vi "SAC-Read Responses.vi"(2 "State":T1, 7 "filestem":string, 11 "error in (no error)":errorcluster) -> (6 "time":cluster{"offset":dbl, "dx":dbl, "Y":dbl[]}, 8 "crosscorr":cluster{"offset":dbl, "dx":dbl, "Y":dbl[]}, 13 "phase":cluster{"offset":dbl, "dx":dbl, "Y":dbl[]}, 14 "mag":cluster{"offset":dbl, "dx":dbl, "Y":dbl[]}, 15 "error out":errorcluster)   [LabVIEW 2020]
uses:
  Typedefs/SAC-State.ctl
  <vilib>/Analysis/2dsp.llb/Complex FFT.vi
  <vilib>/Analysis/2dsp.llb/Inverse Real FFT.vi
  Utility VIs/Math VIs/FFT x(t) to dB,Degrees (1D).vi
  Utility VIs/Conversion VIs/Create Waveform Cluster (1D).vi
  <vilib>/Analysis/NI_AALPro.lvlib
panel:
  out "error out":errorcluster
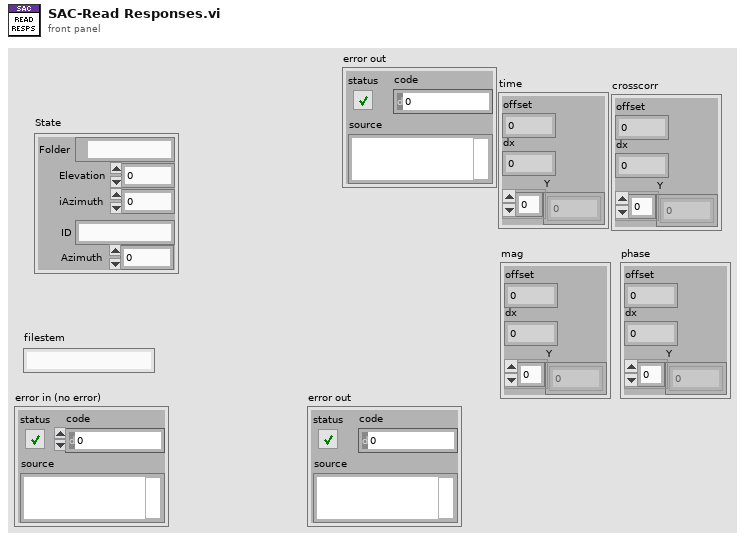
[diagram p1: front panel]
types:
  T1 = typedef "SAC-State.ctl" = cluster{"Folder":path, "Elevation":dbl, "iAzimuth":i32, "ID":string, "Azimuth":dbl}
  T2 = typedef "SAC-Parameters.ctl" = cluster{"Fs (Hz)":dbl, "atten (dB)":dbl, "Waveform":T3, "Freq Res (Hz)":dbl, "Order":i32, "Averages":i32, "seed":i64, "Window":T4, "Mic gain":dbl, "Mic sens":dbl}
  T3 = typedef "HRTF-Waveform.ctl" = enum16{"Chirp", "MLS"}
  T4 = typedef "HRTF-Window.ctl" = cluster{"Type":T5, "Length (ms)":dbl, "Center (ms)":dbl}
  T5 = typedef "HRTF-Window Type.ctl" = enum16{"None", "Rectangle", "Hanning"}
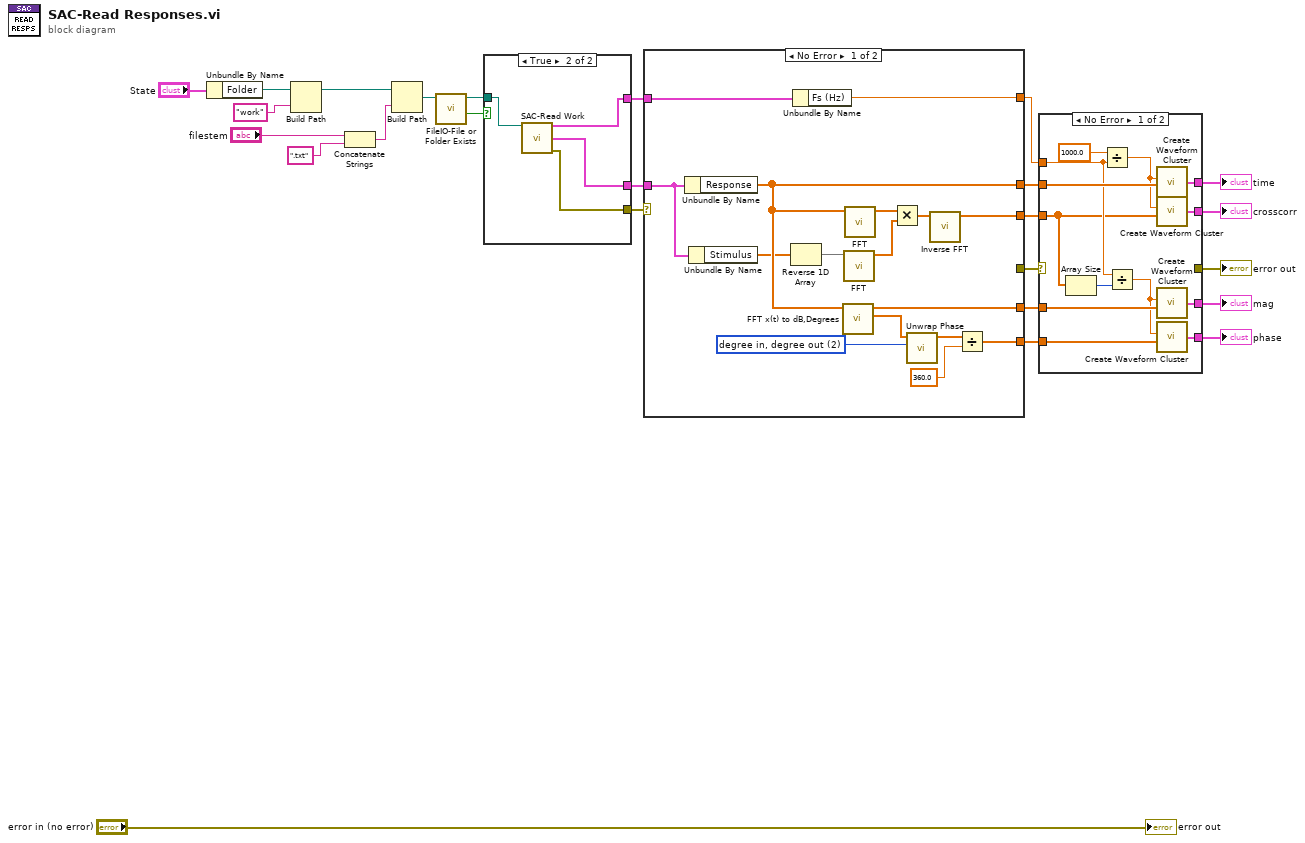
[diagram p0: block diagram]
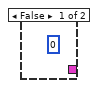
[diagram p2: hidden frame]
diagram:
  n1 = Unbundle By Name("State") -> ("Folder"=w23:path)
  n2 = Build Path(base path=w23, name or relative path="work") -> (appended path=w10:path)
  n3 = Concatenate Strings("filestem", ".txt" ("format string")) -> (w1:string)
  n4 = Build Path(base path=w10, name or relative path=w1) -> (appended path=w6:path)
  n5 = call "FileIO-File or Folder Exists.vi"("path"=w6) -> ("Exists?"=w4:bool, "dup path"=w5:path)  [unwired: 7 in, 2 out]
  n6 = case shown="True" w4 {
    tunnel: [_ w27] -> w8
    tunnel: w5 -> [_ w29]
    tunnel: [_ w26] -> w21
    tunnel: [_ w28] -> w22
    frame False {
      (unwired) 0
    }
    frame True {
      n7 = call "SAC-Read Work.vi"("path"=w29) -> ("Params"=w27:T2, "Result"=w26:cluster{"Stimulus":dbl[], "Response":dbl[]}, "error out"=w28:errorcluster)  [unwired: 12 in]
    }
  }
  n8 = case shown="No Error" w22 {
    selector: w22 -> [_ w46]
    tunnel: w21 -> [w45 _]
    tunnel: [_ w46] -> w20
    tunnel: [w44 _] -> w18
    tunnel: [w43 _] -> w19
    tunnel: [w42 _] -> w17
    tunnel: [w41 _] -> w16
    tunnel: w8 -> [w40 _]
    tunnel: [w39 _] -> w7
    frame No Error {
      w36 = 2 items=["radian in, radian out", "radian in, degree out", "degree in, degree out", "degree in, radian out"] ("phase unit")
      n9 = Unbundle By Name(w45) -> ("Response"=w44:dbl[])
      n10 = Unbundle By Name(w45) -> ("Stimulus"=w33:dbl[])
      n11 = Reverse 1D Array(array=w33) -> (reversed array=w34:dbl[])
      n12 = Unbundle By Name(w40) -> ("Fs (Hz)"=w39:dbl)
      n13 = call-poly "FFT x(t) to dB,Degrees.vi"("X"=w44) -> ("+Freq Phase of FFT (degrees)"=w37:dbl[], "+Freq. Mag of FFT (dB rms)"=w42:dbl[])  [unwired: 8 in, 1 out]
      n14 = call-poly <vilib>:"FFT.vi"("X"=w34) -> ("FFT {X}"=w35:cdb[])  [unwired: 9 in, 1 out]
      n15 = call-poly <vilib>:"FFT.vi"("X"=w44) -> ("FFT {X}"=w32:cdb[])  [unwired: 9 in, 1 out]
      n16 = Multiply(x=w32, y=w35) -> (x*y=w31:cdb[])
      n17 = call <vilib>:"Unwrap Phase.vi"("phase unit"=w36, "Phase"=w37) -> ("Unwrapped Phase"=w38:dbl[])  [unwired: 8 in, 1 out]
      n18 = call-poly <vilib>:"Inverse FFT.vi"("FFT {X}"=w31) -> ("X"=w43:dbl[])  [unwired: 9 in, 1 out]
      n19 = Divide(x=w38, y=360.0) -> (x/y=w41:dbl[])
    }
    frame Error {
    }
  }
  n20 = case shown="No Error" w20 {
    selector: w20 -> [_ w60]
    tunnel: w19 -> [w48 _]
    tunnel: w18 -> [w59 _]
    tunnel: w17 -> [w58 _]
    tunnel: w16 -> [w57 _]
    tunnel: [w56 _] -> w15
    tunnel: [w55 _] -> w14
    tunnel: [w54 _] -> w13
    tunnel: [w53 _] -> w12
    tunnel: [_ w60] -> w11
    tunnel: w7 -> [w50 _]
    frame No Error {
      n21 = Array Size(array=w48) -> (size(s)=w47:i32)
      n22 = Divide(x=1000.0, y=w50) -> (x/y=w51:dbl)
      n23 = Divide(x=w50, y=w47) -> (x/y=w49:dbl)
      n24 = call-poly "Create Waveform Cluster.vi"("dx"=w51, "Y"=w59) -> ("waveform cluster"=w56:cluster{dbl, "dx":dbl, "Y":dbl[]})  [unwired: 3 in]
      n25 = call-poly "Create Waveform Cluster.vi"("dx"=w51, "Y"=w48) -> ("waveform cluster"=w55:cluster{dbl, "dx":dbl, "Y":dbl[]})  [unwired: 3 in]
      n26 = call-poly "Create Waveform Cluster.vi"("dx"=w49, "Y"=w58) -> ("waveform cluster"=w54:cluster{dbl, "dx":dbl, "Y":dbl[]})  [unwired: 3 in]
      n27 = call-poly "Create Waveform Cluster.vi"("dx"=w49, "Y"=w57) -> ("waveform cluster"=w53:cluster{dbl, "dx":dbl, "Y":dbl[]})  [unwired: 3 in]
    }
    frame Error {
    }
  }
  "time" <- w15
  "mag" <- w13
  "phase" <- w12
  "crosscorr" <- w14
  "error out" <- w11
  "error out" <- "error in (no error)"
